vi "Calculate Waveform Subset for Measurement.vi"(6 "sampling rate":dbl, 7 "signal frequency":dbl, 8 "minimum settling duration":dbl, 9 "minimum settling cycles":u32, 10 "minimum measurement duration":dbl, 11 "minimum measurement cycles":u32) -> (1 "duration (samples)":u32, 2 "start (samples)":u32, 3 "total acquisition (samples)":u32)   [LabVIEW 2023]
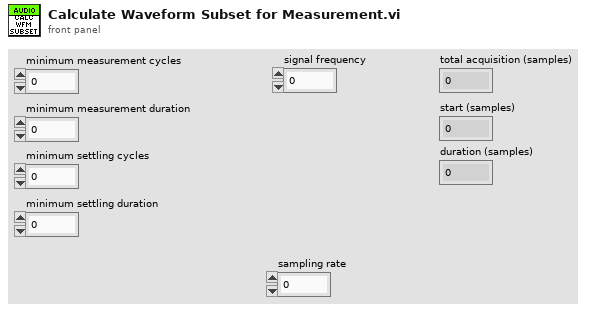
[diagram p1: front panel]
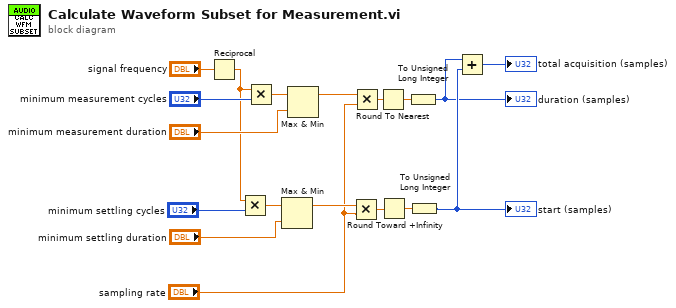
[diagram p0: block diagram]
diagram:
  n1 = Reciprocal(x="signal frequency") -> (1/x=w13:dbl)
  n2 = Multiply(x=w13, y="minimum settling cycles") -> (x*y=w14:dbl)
  n3 = Multiply(x=w13, y="minimum measurement cycles") -> (x*y=w17:dbl)
  n4 = Max & Min(x=w14, y="minimum settling duration") -> (max(x,y)=w12:dbl)  [unwired: 1 out]
  n5 = Max & Min(x=w17, y="minimum measurement duration") -> (max(x,y)=w11:dbl)  [unwired: 1 out]
  n6 = Multiply(x=w12, y="sampling rate") -> (x*y=w6:dbl)
  n7 = Multiply(x=w11, y="sampling rate") -> (x*y=w2:dbl)
  n8 = Round To Nearest(number=w2) -> (nearest integer value=w3:dbl)
  n9 = Round Toward +Infinity(x=w6) -> (ceil(x): smallest int >= x=w5:dbl)
  n10 = To Unsigned Long Integer(number=w3) -> (unsigned 32bit integer=w1:u32)
  "duration (samples)" <- w1
  n11 = To Unsigned Long Integer(number=w5) -> (unsigned 32bit integer=w4:u32)
  "start (samples)" <- w4
  n12 = Add(x=w1, y=w4) -> (x+y=→"total acquisition (samples)":u32)
